vi "AlliGator Python Plugin Valid Output Destination.vi"(2 "Output Destination":string) -> (7 "Valid Destination?":bool)   [LabVIEW 2021, in "AlliGator Python Plugins.lvlib"]
doc: "Checks whether the output destination is valid."
uses:
  AlliGator Python Plugins.lvlib
  Strings/Strings.lvlib
panel:
  # "see the AlliGator License on the block diagram (Ctrl+E or Window:Show Block Diagram)"
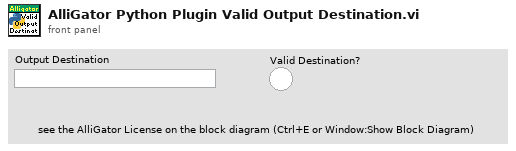
[diagram p1: front panel]
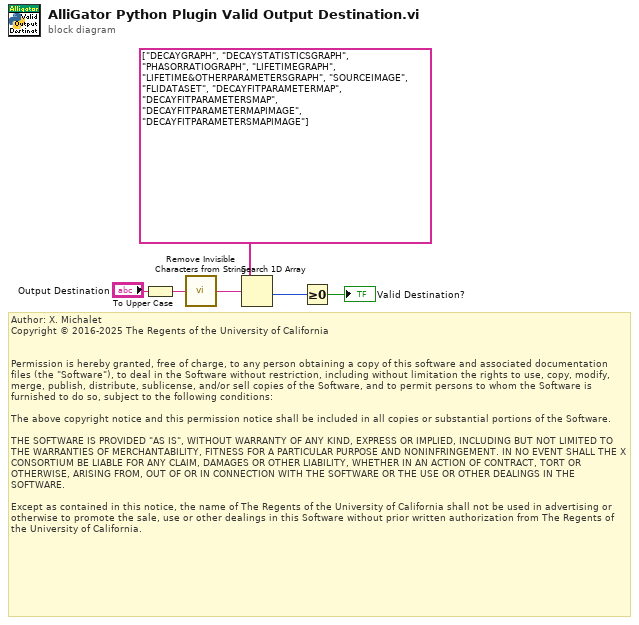
[diagram p0: block diagram]
diagram:
  # "Author: X. Michalet\nCopyright © 2016-2025 The Regents of the University of California\n \n\nPermission is hereby granted, free of charge, to any person obtaining a copy of this software and associated documentation files (the \"Software\"), to deal in the Software without restriction, including without limitation the rights to use, copy, modify, merge, publish, distribute, sublicense, and/or sell copies of the Software, and to permit persons to whom the Software is furnished to do so, subject to the following conditions:\n\nThe above copyright notice and this permission notice shall be included in all copies or substantial portions of the Software.\n\nTHE SOFTWARE IS PROVIDED \"AS IS\", WITHOUT WARRANTY OF ANY KIND, EXPRESS OR IMPLIED, INCLUDING BUT NOT LIMITED TO THE WARRANTIES OF MERCHANTABILITY, FITNESS FOR A PARTICULAR PURPOSE AND NONINFRINGEMENT. IN NO EVENT SHALL THE X CONSORTIUM BE LIABLE FOR ANY CLAIM, DAMAGES OR OTHER LIABILITY, WHETHER IN AN ACTION OF CONTRACT, TORT OR OTHERWISE, ARISING FROM, OUT OF OR IN CONNECTION WITH THE SOFTWARE OR THE USE OR OTHER DEALINGS IN THE SOFTWARE.\n\nExcept as contained in this notice, the name of The Regents of the University of California shall not be used in advertising or otherwise to promote the sale, use or other dealings in this Software without prior written authorization from The Regents of the University of California."
  n1 = To Upper Case(1:"Output Destination") -> (0:w4:string)
  n2 = call "Remove Invisible Characters from String.vi"("String"=w4) -> ("result string"=w1:string)  [unwired: 3 in]
  n3 = Search 1D Array(1D array=string[] ["DECAYGRAPH", "DECAYSTATISTICSGRAPH", "PHASORRATIOGRAPH", "LIFETIMEGRAPH", "LIFETIME&OTHERPARAMETERSGRAPH", "SOURCEIMAGE", "FLIDATASET", "DECAYFITPARAMETERMAP", "DECAYFITPARAMETERSMAP", "DECAYFITPARAMETERMAPIMAGE", "DECAYFITPARAMETERSMAPIMAGE"], element=w1) -> (index of element=w3:i32)  [unwired: 1 in]
  n4 = Greater Or Equal To 0?(x=w3) -> (x >= 0?=→"Valid Destination?":bool)
